vi "Handle Value Changed.vi"(6 "dValue":dbl, 8 "error in":errorcluster, 9 "Control Ref":refnum<k24>, 10 "Event Common Data":T1, 11 "MyEventGrid in":refnum<class "MyEventGrid.lvclass">) -> (0 "error out":errorcluster, 3 "MyEventGrid out":refnum<class "MyEventGrid.lvclass">)   [LabVIEW 2024, in "MyEventGrid.lvclass"]
uses:
  MyEventGrid.lvclass
  C:/Program Files/National Instruments/LabVIEW 2024/examples/Connectivity/Dot NET/EventExample.dll
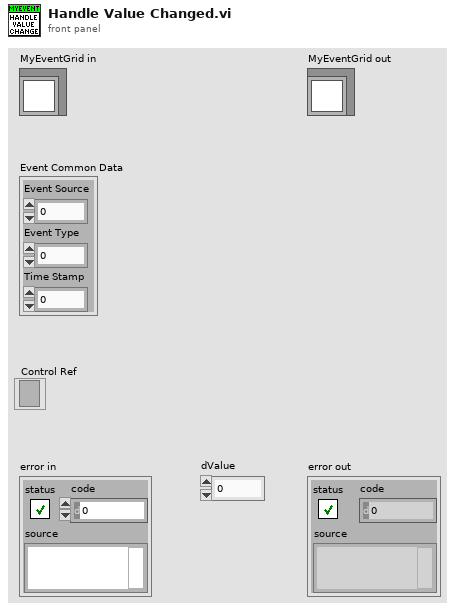
[diagram p1: front panel]
types:
  T1 = cluster{"Event Source":i32, "Event Type":u32, "Time Stamp":u32}
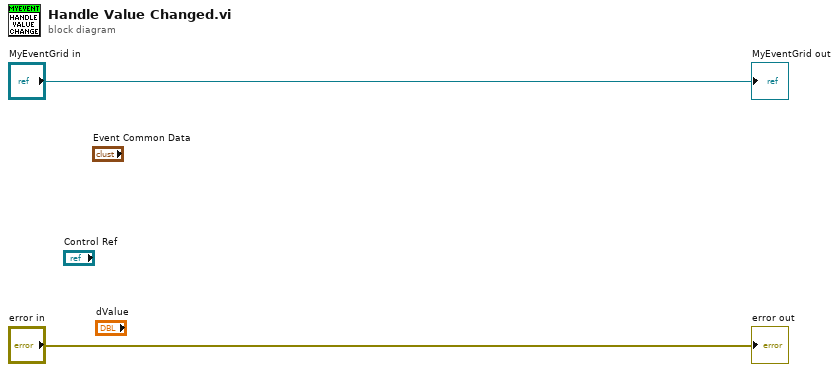
[diagram p0: block diagram]
diagram:
  "error out" <- "error in"
  "MyEventGrid out" <- "MyEventGrid in"
